vi "LabVIEW 4 MiniGen_Adafruit.vi"(3 "error in (no error)":errorcluster, 4 "dt":dbl=2.65925481e-05 format="%#_9f", 5 "write buffer":string="r512") -> (0 "error out":errorcluster, 1 "Peak Frequency":dbl=514.1242933391554, 2 "magnitude":cluster{"f0":dbl, "df":dbl, "magnitude":dbl[]}={"f0"=146.89265523975868, "df"=73.44632761987934, "magnitude"=[0.0010573193272467023, 0.0008539075571475185, 0.0031903245438082524, 0.016955292518775398, 0.23690823513289183, 0.3602537891013049, 0.13311105968536813, 0.008147783611046596, 0.0029630449976908928, 0.0006136557806143884, 0.0009534776069795952, 0.0014653745421584592, 0.0018598328245117294, 0.000343909019222686, 0.00033893535263468947, 0.0003721335616413998, 0.0003311608729031368, 0.000732767453399492, 0.001587238767052589, 0.0015399953791484678, 0.0006799804044090185, 0.00035922580059501353, 0.00037853640587946584, 0.00040574798016109284, 0.0003944657918505259, 0.00028441301720993916, 0.000261065277392889, 9.830660293093549e-05, 0.00043397339336911814, 0.0005539762634671169, 0.00040990403678268047, 0.00029319183108519875, 8.368304059100074e-05, 8.36004681704598e-05, 0.00015879910796170698, 6.252358099316568e-05, 0.00015881977208714157, 0.00016509561428111567, 6.434491581170871e-05, 0.0001668647295604266, 0.00036578961819133, 0.00045765208783560507, 0.0005154983450355664, 0.0005172148246027255, 0.0003062574513331491, 5.1513455854055797e-05, 0.00023831181783032655, 0.00024374499609663026, 0.0001419110455078641, 0.00041264635419791494, 0.00022761885947105454, 0.00038244224659812054, 0.0003878354411526907, 0.0003434041323071504, 0.00035602580591923087, 0.0003014195763820755, 0.00010701693781615192, 0.00016376183360085065, 0.00021830596775413067, 0.0004512016989735132, 0.00038858135278494886, 0.0003582381020895125, 0.00015397417992981166, 0.00025184195021753214, 0.0003101067745655077, 0.000447806893819167, 0.0006303208430332876, 0.0005244485053927753, 0.0003894931417183425, 0.0002169168936988449, 0.00015424488539364647, 7.28953873783167e-05, 0.00015840874717917624, 0.00030123326854442566, 0.0003357070951253949, 0.0002219813177305886, 2.7096544974727197e-05, 3.534450755456907e-05, 3.428286160556027e-05, 0.00024763168162031965, 0.0005956370452363904, 0.0005001341365814027, 0.0002493340489535057, 8.913553682671315e-05, 4.102695129838161e-05, 0.00023937047150089836, 0.0006064155727417735, 0.0007636718971057465, 0.0005025169233197376, 0.0004592141713891292, 0.0004154038880786475, 0.0004762512230483866, 0.00032394851279825726, 0.00019874656152786516, 0.00024103234975927565, 0.00024679552700484163, 0.00022974190446812425, 0.00014852727721558983, 0.0001534539800413088, 0.0002623950929260538, 0.00020502102196828442, 2.0769438374928514e-05, 3.7831709687521644e-05, 0.00016600027554920273, 7.477285742547296e-05, 0.00015424772258269823, 0.00014615356739457614, 0.0005738937352417223, 0.0005461816457255241, 0.00043653069066669405, 0.00044891438828865895, 0.00033415133284021457, 0.0004333097052614254, 0.0005465034873180447, 0.0004401723358116891, 0.0003491099907256788, 0.00034433390816092396, 0.0001621270437531999, 0.0003023179218436354, 0.000471682669669569, 0.00024159641785356876, 7.693286124485976e-05, 0.0002467093051980444, 0.0003294163904248798, 0.0003712395660317976, 0.00025510195803937145, 0.0002820556822567327, 0.00026127126859739616, 0.0004117321530064503, 0.00026155711305912867, 0.0003954869452259379, 0.0005027179953043017, 0.0002034553573790203, 0.00031739709370906294, 0.000494844481482639, 0.0003194082061686813, 0.00017347199605366486, 0.00030810211276043666, 0.00019142967321880493, 9.299614747889054e-05, 0.00022546314931713994, 0.00024526204479037166, 0.0003803466725698766, 0.0005482171928358633, 0.00022244146310983445, 8.882750051753354e-05, 0.0001521589339551093, 6.025891276057421e-05, 0.00010936756826677184, 0.00011678105621078553, 0.00027208101011661, 0.0003853539959161425, 0.00019733124731021647, 0.0002399298595306906, 0.0003751773029308181, 0.00025934156594460743, 0.0003897060735522648, 0.00028379388433385095, 0.00017344162601981542, 8.946407319767827e-05, 0.0002479505393338664, 0.00027803060344221684, 0.00021717165064423773, 0.0002199029505972962, 0.0004957184252712735, 0.0004894240536570223, 0.0002533586709072349, 0.0001130558253712342, 0.0002151253256980126, 0.00025783922831527315, 8.558793567000533e-05, 0.00023749246624682629, 8.271720418254696e-05, 0.00019562076852570315, 0.00022269512667799665, 0.0002276244107757865, 0.0002727820351925076, 0.00039997710573542355, 0.00032310482776941204, 0.00029355353878777286, 6.098205313979909e-05, 0.0002335475568675092, 0.00016341841260641903, 0.00022823089080733973, 0.0003044010656702124, 0.0001623398261568934, 0.0004701790442476819, 0.0004588133187804099, 0.0006269691947846191, 0.0005404430387144859, 0.00040211372693186285, 0.00019372670536392075, 6.440168512958198e-05, 0.00025538585629209166, 0.0002603927600912937, 0.00025560577048397464, 0.0002262629957829637, 0.0003607957498107714, 0.00030784688204000616, 0.00021197768635284272, 0.0003775437438451099, 0.0002709208729009615, 7.259587758192056e-05, 0.00042224897133781364, 0.0007178070922026255, 0.00047376015823390833, 0.0002390419285937669, 0.00041521474238425424, 0.000549847037281132, 0.00039822948997910514, 0.00044424119183215043, 0.00028924976182143454, 0.000392533131171722, 0.0006030596886870012, 0.00042943037291800384, 0.00015018445254512435, 0.0003089247263095562, 0.00042702952337648293, 0.0003129672107102853, 0.00022654935544524929, 0.00016456577793551, 0.00038796014465995233, 0.00021047618867833676, 0.0002206211444044933, 0.00035334155895193125, 0.00019866739041272719, 0.0002668159983142619, 0.0004925200936011109, 0.00037262502516944185, 0.0003256045216749679, 0.0003440845270831269, 0.0001665288519916862, 0.0001746740042938917, 0.00036685704356912417, 0.0003280980682345908, 0.00026309028815703155, 0.00026930545946579566, 0.000340611458947099, 0.0003731069571000136, 0.0002468870659088116, 0.0002756449502200578, 0.00035429030046231887, 0.0003621555052894118, 0.0003683074149373423, 0.0003306130216987354, 0.00023802697854053423, 8.317737651327105e-05, 0.00015097842581436664, 0.0003288513395746616, 7.503484674742626e-05, 0.00012634741676269078, 6.831559096065801e-05, 0.00020546353367269728, 0.0002085374736113191]} {"magnitude" format="%.2p"; "f0" format="%0.2p"; "df" format="%0.2p"})   [LabVIEW 2020]
uses:
  <vilib>/Instr/_visa.llb/VISA Flush IO Buffer Mask.ctl
  <vilib>/Instr/_visa.llb/VISA Configure Serial Port (Instr).vi
  <vilib>/measure/maspectr.llb/FFT Spectrum (Mag-Phase) for 1 Chan.vi
  <vilib>/measure/NI_MAPro.lvlib
panel:
  in  "Base Freq":dbl=210.0
  out "New Freqency":dbl=11319170.442154845 format="%#_10f"
  in  "N":i32=301
  out "Sample Rate":dbl=37604.51974137822
  out "Waveform Graph":cluster{"f0":dbl, "df":dbl, "magnitude":dbl[]}(graph)={"f0"=146.89265523975868, "df"=73.44632761987934, "magnitude"=[0.0010573193272467023, 0.0008539075571475185, 0.0031903245438082524, 0.016955292518775398, 0.23690823513289183, 0.3602537891013049, 0.13311105968536813, 0.008147783611046596, 0.0029630449976908928, 0.0006136557806143884, 0.0009534776069795952, 0.0014653745421584592, 0.0018598328245117294, 0.000343909019222686, 0.00033893535263468947, 0.0003721335616413998, 0.0003311608729031368, 0.000732767453399492, 0.001587238767052589, 0.0015399953791484678, 0.0006799804044090185, 0.00035922580059501353, 0.00037853640587946584, 0.00040574798016109284, 0.0003944657918505259, 0.00028441301720993916, 0.000261065277392889, 9.830660293093549e-05, 0.00043397339336911814, 0.0005539762634671169, 0.00040990403678268047, 0.00029319183108519875, 8.368304059100074e-05, 8.36004681704598e-05, 0.00015879910796170698, 6.252358099316568e-05, 0.00015881977208714157, 0.00016509561428111567, 6.434491581170871e-05, 0.0001668647295604266, 0.00036578961819133, 0.00045765208783560507, 0.0005154983450355664, 0.0005172148246027255, 0.0003062574513331491, 5.1513455854055797e-05, 0.00023831181783032655, 0.00024374499609663026, 0.0001419110455078641, 0.00041264635419791494, 0.00022761885947105454, 0.00038244224659812054, 0.0003878354411526907, 0.0003434041323071504, 0.00035602580591923087, 0.0003014195763820755, 0.00010701693781615192, 0.00016376183360085065, 0.00021830596775413067, 0.0004512016989735132, 0.00038858135278494886, 0.0003582381020895125, 0.00015397417992981166, 0.00025184195021753214, 0.0003101067745655077, 0.000447806893819167, 0.0006303208430332876, 0.0005244485053927753, 0.0003894931417183425, 0.0002169168936988449, 0.00015424488539364647, 7.28953873783167e-05, 0.00015840874717917624, 0.00030123326854442566, 0.0003357070951253949, 0.0002219813177305886, 2.7096544974727197e-05, 3.534450755456907e-05, 3.428286160556027e-05, 0.00024763168162031965, 0.0005956370452363904, 0.0005001341365814027, 0.0002493340489535057, 8.913553682671315e-05, 4.102695129838161e-05, 0.00023937047150089836, 0.0006064155727417735, 0.0007636718971057465, 0.0005025169233197376, 0.0004592141713891292, 0.0004154038880786475, 0.0004762512230483866, 0.00032394851279825726, 0.00019874656152786516, 0.00024103234975927565, 0.00024679552700484163, 0.00022974190446812425, 0.00014852727721558983, 0.0001534539800413088, 0.0002623950929260538, 0.00020502102196828442, 2.0769438374928514e-05, 3.7831709687521644e-05, 0.00016600027554920273, 7.477285742547296e-05, 0.00015424772258269823, 0.00014615356739457614, 0.0005738937352417223, 0.0005461816457255241, 0.00043653069066669405, 0.00044891438828865895, 0.00033415133284021457, 0.0004333097052614254, 0.0005465034873180447, 0.0004401723358116891, 0.0003491099907256788, 0.00034433390816092396, 0.0001621270437531999, 0.0003023179218436354, 0.000471682669669569, 0.00024159641785356876, 7.693286124485976e-05, 0.0002467093051980444, 0.0003294163904248798, 0.0003712395660317976, 0.00025510195803937145, 0.0002820556822567327, 0.00026127126859739616, 0.0004117321530064503, 0.00026155711305912867, 0.0003954869452259379, 0.0005027179953043017, 0.0002034553573790203, 0.00031739709370906294, 0.000494844481482639, 0.0003194082061686813, 0.00017347199605366486, 0.00030810211276043666, 0.00019142967321880493, 9.299614747889054e-05, 0.00022546314931713994, 0.00024526204479037166, 0.0003803466725698766, 0.0005482171928358633, 0.00022244146310983445, 8.882750051753354e-05, 0.0001521589339551093, 6.025891276057421e-05, 0.00010936756826677184, 0.00011678105621078553, 0.00027208101011661, 0.0003853539959161425, 0.00019733124731021647, 0.0002399298595306906, 0.0003751773029308181, 0.00025934156594460743, 0.0003897060735522648, 0.00028379388433385095, 0.00017344162601981542, 8.946407319767827e-05, 0.0002479505393338664, 0.00027803060344221684, 0.00021717165064423773, 0.0002199029505972962, 0.0004957184252712735, 0.0004894240536570223, 0.0002533586709072349, 0.0001130558253712342, 0.0002151253256980126, 0.00025783922831527315, 8.558793567000533e-05, 0.00023749246624682629, 8.271720418254696e-05, 0.00019562076852570315, 0.00022269512667799665, 0.0002276244107757865, 0.0002727820351925076, 0.00039997710573542355, 0.00032310482776941204, 0.00029355353878777286, 6.098205313979909e-05, 0.0002335475568675092, 0.00016341841260641903, 0.00022823089080733973, 0.0003044010656702124, 0.0001623398261568934, 0.0004701790442476819, 0.0004588133187804099, 0.0006269691947846191, 0.0005404430387144859, 0.00040211372693186285, 0.00019372670536392075, 6.440168512958198e-05, 0.00025538585629209166, 0.0002603927600912937, 0.00025560577048397464, 0.0002262629957829637, 0.0003607957498107714, 0.00030784688204000616, 0.00021197768635284272, 0.0003775437438451099, 0.0002709208729009615, 7.259587758192056e-05, 0.00042224897133781364, 0.0007178070922026255, 0.00047376015823390833, 0.0002390419285937669, 0.00041521474238425424, 0.000549847037281132, 0.00039822948997910514, 0.00044424119183215043, 0.00028924976182143454, 0.000392533131171722, 0.0006030596886870012, 0.00042943037291800384, 0.00015018445254512435, 0.0003089247263095562, 0.00042702952337648293, 0.0003129672107102853, 0.00022654935544524929, 0.00016456577793551, 0.00038796014465995233, 0.00021047618867833676, 0.0002206211444044933, 0.00035334155895193125, 0.00019866739041272719, 0.0002668159983142619, 0.0004925200936011109, 0.00037262502516944185, 0.0003256045216749679, 0.0003440845270831269, 0.0001665288519916862, 0.0001746740042938917, 0.00036685704356912417, 0.0003280980682345908, 0.00026309028815703155, 0.00026930545946579566, 0.000340611458947099, 0.0003731069571000136, 0.0002468870659088116, 0.0002756449502200578, 0.00035429030046231887, 0.0003621555052894118, 0.0003683074149373423, 0.0003306130216987354, 0.00023802697854053423, 8.317737651327105e-05, 0.00015097842581436664, 0.0003288513395746616, 7.503484674742626e-05, 0.00012634741676269078, 6.831559096065801e-05, 0.00020546353367269728, 0.0002085374736113191]}
  in  "VISA resource name":refnum<visa-resource-name>="COM12"
  out "read buffer":string="Output = 2500,2454,2418,2378,2328,2280,2224,2162,2104,2066,2008,1948,1896,1840,1788,1742,1694,1660,1616,1584,1540,1510,1486,1468,1448,1438,1426,1422,1428,1420,1432,1456,1468,1486,1504,1548,1582,1620,1648,1702,1748,1788,1850,1896,1954,1988,2044,2110,2170,2218,2272,2320,2368,2412,2468,2506,2530,2576,2598,2628,2662,2676,2684,2698,2712,2714,2716,2710,2694,2684,2664,2644,2618,2580,2558,2510,2472,2432,2388,2334,2288,2226,2186,2124,2076,2014,1960,1916,1860,1808,1764,1706,1670,1630,1590,1556,1520,1492,1476,1450,1448,1426,1418,1426,1424,1430,1442,1468,1482,1506,1540,1572,1602,1644,1690,1736,1788,1836,1886,1934,1996,2044,2096,2150,2210,2260,2304,2354,2410,2454,2500,2530,2568,2598,2628,2660,2666,2694,2694,2710,2710,2704,2710,2694,2674,2656,2644,2612,2590,2556,2510,2476,2426,2382,2344,2290,2238,2186,2130,2082,2010,1956,1916,1852,1814,1754,1718,1672,1628,1596,1562,1520,1496,1478,1460,1446,1432,1424,1428,1414,1432,1452,1456,1474,1504,1538,1558,1600,1638,1682,1726,1774,1828,1870,1916,1966,2030,2090,2138,2192,2254,2288,2348,2384,2436,2488,2516,2550,2592,2626,2650,2664,2684,2700,2706,2716,2714,2704,2694,2680,2664,2656,2626,2600,2570,2528,2484,2452,2398,2362,2306,2260,2206,2144,2100,2042,1986,1942,1878,1830,1776,1722,1686,1632,1606,1570,1536,1500,1482,1466,1442,1430,1430,1414,1428,1428,1444,1454,1474,1498,1512,1564,1582,1620,1652,1706,1760,1810,1862,1902,1960,2022,2082,2134,2186,2238,2288,2342,2388,2428,2480,2522,2548,2592,2622,2648,2660,2674,2686,2712,2714,2718,2702,2694,2696,2672,2648,2628,2612,2572,2532,2500,2460,2422,2372,2320,2272,2218,2162,2106,2048,1998,1942,1886,1830,1776,1740,1690,1650,1614,1572,1546,1502,1490,1460,1444,1434,1426,1426,1428,1424,1436,1456,1462,1488,1522,1556,1578,1624,1664,1712,1758,1796,1848,1900,1950,2014,2072,2116,2182,2234,2278,2334,2374,2434,2472,2514,2552,2582,2618,2634,2660,2674,2688,2696,2700,2718,2704,2706,2694,2668,2658,2636,2604,2566,2534,2494,2466,2420,2370,2314,2264,2218,2172,2106,2062,1998,1948,1898,1848,1794,1742,1696,1650,1616,1574,1546,1514,1486,1464,1452,1440,1424,1420,1416,1432,1440,1448,1464,1482,1518,1542,1580,1612,1652,1706,1748,1806,1856,1894,1958,2010,2062,2116,2180,2232,2286,2330,2384,2428,2474,2510,2554,2588,2616,2640,2666,2680,2684,2698,2716,2708,2712,2706,2694,2676,2648,2624,2604,2578,2538,2492,2460,2414,2368,2326,2266,2206,2158,2104,2062,1992,1940,1892,1838,1792,1736,1700,1652,1616,1578,1546,1518,1492,1454,1454,1428,1432,1432,1412,1430,1434,1444,1472,1494,1522,1550,1574,1620,1662,1696,1748,1796,1852,1900,1950,2004,2062,2122,2174,2226,2274,2328,2372,2416,2462,2506,2548,2584,2604,2638,2660\r\n"
  out "XY Graph":cluster{dbl[], dbl[]}[](graph)
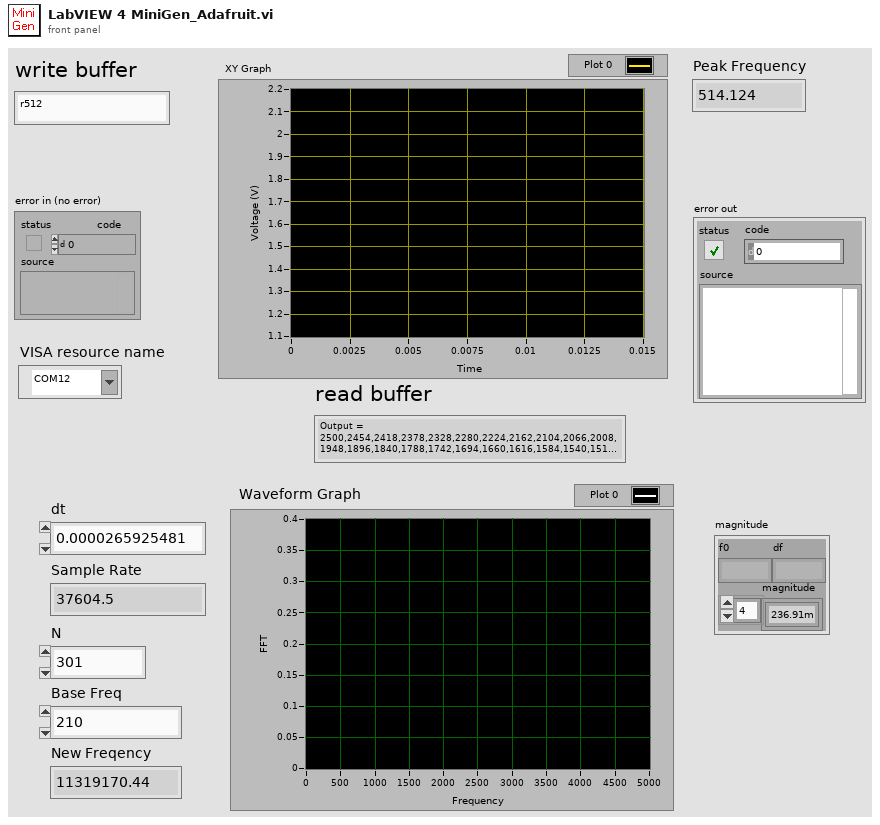
[diagram p1: front panel]
types:
  T1 = typedef "VISA Flush IO Buffer Mask.ctl" = u16
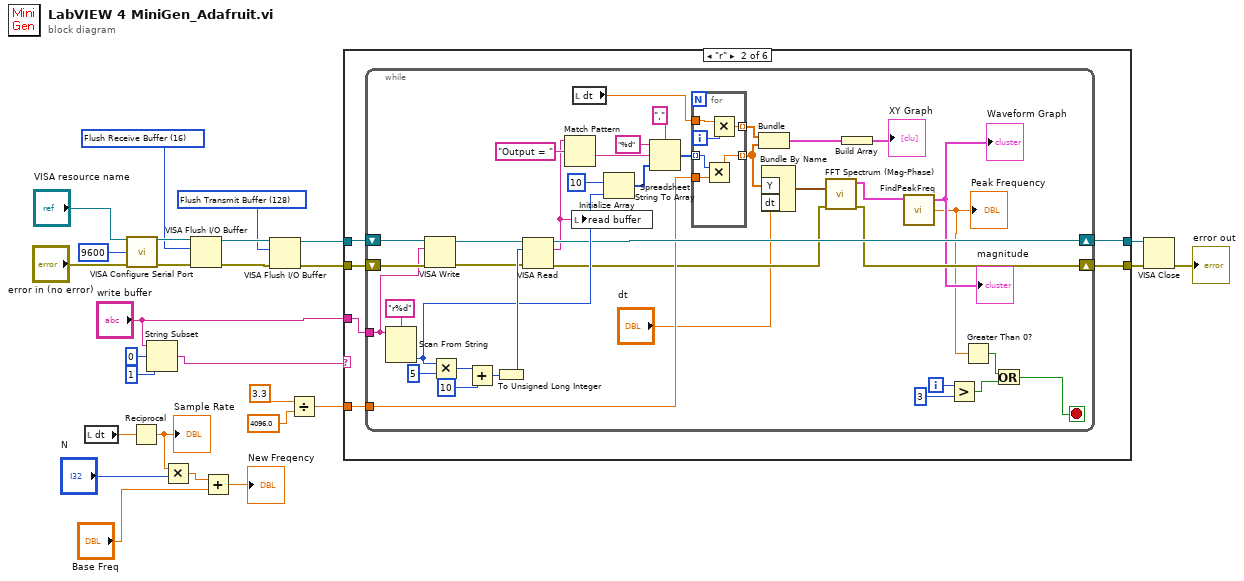
[diagram p0: block diagram]
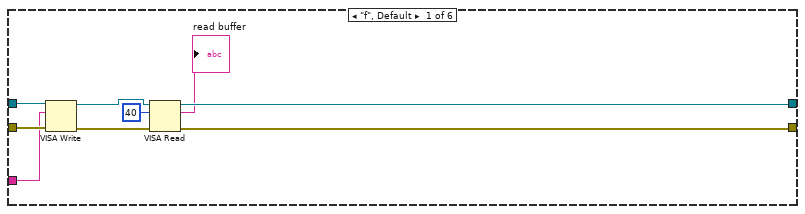
[diagram p2: hidden frame]
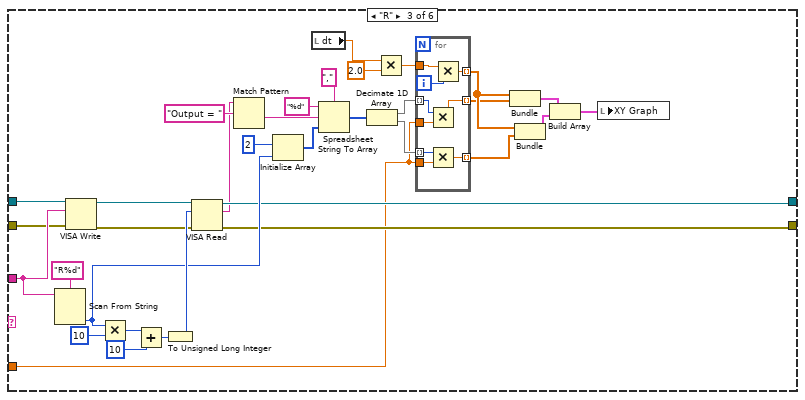
[diagram p3: hidden frame]
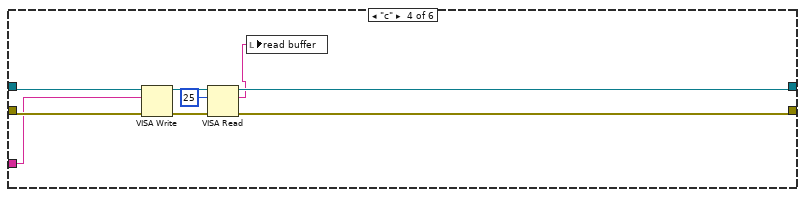
[diagram p4: hidden frame]
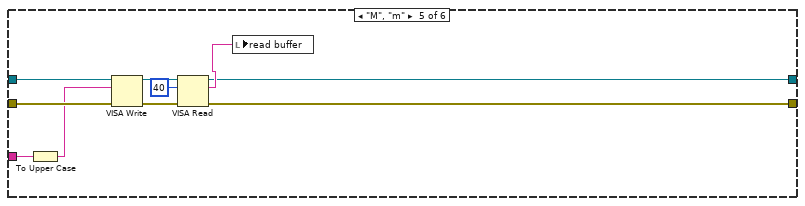
[diagram p5: hidden frame]
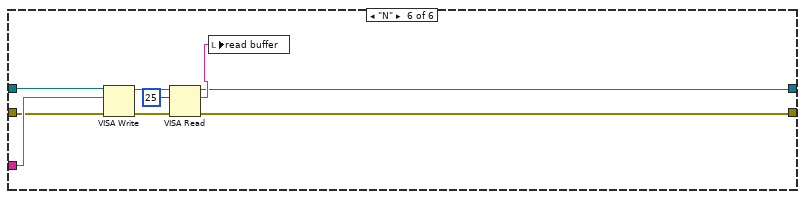
[diagram p6: hidden frame]
diagram:
  w21 = T1 128 items=["Flush Receive Buffer"=16, "Write Transmit Buffer to Device"=32, "Flush Receive Buffer (No I/O)"=64, "Flush Transmit Buffer"=128] ("Mask")
  w24 = T1 16 items=["Flush Receive Buffer"=16, "Write Transmit Buffer to Device"=32, "Flush Receive Buffer (No I/O)"=64, "Flush Transmit Buffer"=128] ("Mask")
  n1 = local read "dt"() -> (w8:dbl)
  n2 = call-poly "VISA Configure Serial Port"("VISA resource name"="VISA resource name", "baud rate (9600)"=u32 9600, "error in (no error)"="error in (no error)") -> ("VISA resource name out"=w26:refnum<visa-resource-name>, "error out"=w25:errorcluster)  [unwired: 11 in]
  n3 = Reciprocal(x=w8) -> (1/x=w7:dbl)
  "Sample Rate" <- w7
  n4 = String Subset(string="write buffer", offset (0)=0, length (rest)=1 ("length (rest)")) -> (substring=w14:string)
  n5 = Multiply(x=w7, y="N") -> (x*y=w5:dbl)
  n6 = VISA Flush I/O Buffer(VISA resource name=w26, mask (16)=w24, error in (no error)=w25) -> (VISA resource name out=w23:refnum<visa-resource-name>, error out=w22:errorcluster)
  n7 = Add(x=w5, y="Base Freq") -> (x+y=→"New Freqency":dbl)
  n8 = VISA Flush I/O Buffer(VISA resource name=w23, mask (16)=w21, error in (no error)=w22) -> (VISA resource name out=w2:refnum<visa-resource-name>, error out=w1:errorcluster)
  n9 = Divide(x=3.3, y=4096.0) -> (x/y=w9:dbl)
  n10 = case shown="\"r\"" w14 {
    tunnel: [w36 w37 w106 w133 w140 w150] -> w20
    tunnel: [w34 w39 w107 w134 w141 w151] -> w19
    tunnel: w2 -> [w32 w41 w95 w136 w145 w154]
    tunnel: w1 -> [w31 w40 w93 w135 w144 w152]
    tunnel: "write buffer" -> [w28 w42 w94 w132 w143 w153]
    tunnel: w9 -> [_ w38 w98 _ _ _]
    frame "f", Default {
      n11 = VISA Write(VISA resource name=w32, write buffer=w28, error in (no error)=w31) -> (VISA resource name out=w29:refnum<visa-resource-name>, error out=w30:errorcluster)  [unwired: 1 out]
      n12 = VISA Read(VISA resource name=w29, byte count=u32 40, error in (no error)=w30) -> (VISA resource name out=w34:refnum<visa-resource-name>, read buffer=→"read buffer":string, error out=w36:errorcluster)  [unwired: 1 out]
    }
    frame "r" {
      n13 = while {
        tunnel: w42 -> [w50]
        tunnel: w38 -> [w63]
        shift-right: [w64] -> w39
        shift-left: w41 -> [w54]
        shift-right: [w60] -> w37
        shift-left: w40 -> [w53]
        i -> [w48]
        stop <- w44 stop-if-true
        n14 = Scan From String(format string="r%d", input string=w50) -> (output 1=w70:i32)  [unwired: 3 in, 3 out]
        n15 = VISA Write(VISA resource name=w54, write buffer=w50, error in (no error)=w53) -> (VISA resource name out=w51:refnum<visa-resource-name>, error out=w52:errorcluster)  [unwired: 1 out]
        n16 = Multiply(x=w70, y=5) -> (x*y=w79:i32)
        n17 = Add(x=w79, y=10) -> (x+y=w77:i32)
        n18 = To Unsigned Long Integer(number=w77) -> (unsigned 32bit integer=w76:u32)
        n19 = VISA Read(VISA resource name=w51, byte count=w76, error in (no error)=w52) -> (VISA resource name out=w64:refnum<visa-resource-name>, read buffer=w43:string, error out=w61:errorcluster)  [unwired: 1 out]
        n20 = Match Pattern(string=w43, regular expression="Output = ") -> (after substring=w74:string)  [unwired: 1 in, 3 out]
        n21 = local write "read buffer"(w43) -> ()
        n22 = local read "dt"() -> (w58:dbl)
        n23 = Initialize Array(10 ("y"), w70) -> (w69:i32[])
        n24 = Spreadsheet String To Array(delimiter (Tab)=",", format string="%d", spreadsheet string=w74, array type (2D Dbl)=w69) -> (array=w68:i32[])
        n25 = for {
          tunnel: w68 -> [w87] mode=indexing
          tunnel: [w85] -> w57 mode=indexing
          tunnel: [w82] -> w67 mode=indexing
          tunnel: w63 -> [w86]
          tunnel: w58 -> [w83]
          i -> [w84]
          n26 = Multiply(x=w87, y=w86) -> (x*y=w85:dbl)
          n27 = Multiply(x=w83, y=w84) -> (x*y=w82:dbl)
        }
        n28 = Bundle(w67, w57) -> (w66:cluster{dbl[], dbl[]})  [unwired: 1 in]
        n29 = Bundle By Name("Y"=w57, "dt"="dt") -> (w62:waveform(dbl))  [unwired: 1 in]
        n30 = call-poly <vilib>:"FFT Spectrum (Mag-Phase).vi"("error in (no error)"=w61, "time signal"=w62) -> ("error out"=w60:errorcluster, "magnitude"=w56:cluster{"f0":dbl, "df":dbl, "magnitude":dbl[]})  [unwired: 5 in, 3 out]
        n31 = Build Array(w66) -> (→"XY Graph":cluster{dbl[], dbl[]}[])
        n32 = call "FindPeakFreq.vi"("magnitude"=w56) -> ("Max"=w49:dbl, "output cluster"=→"Waveform Graph" →"magnitude":cluster{"f0":dbl, "df":dbl, "magnitude":dbl[]})  [unwired: 3 in]
        "Peak Frequency" <- w49
        n33 = Greater?(x=w48, y=3) -> (0:w46:bool)
        n34 = Greater Than 0?(x=w49) -> (x > 0?=w45:bool)
        n35 = Or(x=w45, y=w46) -> (x .or. y?=w44:bool)
      }
    }
    frame "R" {
      n36 = Scan From String(format string="R%d", input string=w94) -> (output 1=w109:i32)  [unwired: 3 in, 3 out]
      n37 = VISA Write(VISA resource name=w95, write buffer=w94, error in (no error)=w93) -> (VISA resource name out=w92:refnum<visa-resource-name>, error out=w91:errorcluster)  [unwired: 1 out]
      n38 = Multiply(x=w109, y=10) -> (x*y=w119:i32)
      n39 = Add(x=w119, y=10) -> (x+y=w117:i32)
      n40 = To Unsigned Long Integer(number=w117) -> (unsigned 32bit integer=w116:u32)
      n41 = VISA Read(VISA resource name=w92, byte count=w116, error in (no error)=w91) -> (VISA resource name out=w107:refnum<visa-resource-name>, read buffer=w96:string, error out=w106:errorcluster)  [unwired: 1 out]
      n42 = Match Pattern(string=w96, regular expression="Output = ") -> (after substring=w114:string)  [unwired: 1 in, 3 out]
      n43 = Initialize Array(2 ("y"), w109) -> (w111:i32[])
      n44 = local read "dt"() -> (w89:dbl)
      n45 = Spreadsheet String To Array(delimiter (Tab)=",", format string="%d", spreadsheet string=w114, array type (2D Dbl)=w111) -> (array=w108:i32[])
      n46 = Decimate 1D Array(w108) -> (w105:i32[], w104:i32[])
      n47 = Multiply(x=w89, y=2.0) -> (x*y=w90:dbl)
      n48 = for {
        tunnel: w105 -> [w130] mode=indexing
        tunnel: [w128] -> w100 mode=indexing
        tunnel: [w125] -> w101 mode=indexing
        tunnel: w98 -> [w129]
        tunnel: w90 -> [w126]
        tunnel: w104 -> [w124] mode=indexing
        tunnel: [w123] -> w99 mode=indexing
        tunnel: w98 -> [w122]
        i -> [w127]
        n49 = Multiply(x=w130, y=w129) -> (x*y=w128:dbl)
        n50 = Multiply(x=w124, y=w122) -> (x*y=w123:dbl)
        n51 = Multiply(x=w126, y=w127) -> (x*y=w125:dbl)
      }
      n52 = Bundle(w101, w100) -> (w102:cluster{dbl[], dbl[]})  [unwired: 1 in]
      n53 = Bundle(w101, w99) -> (w103:cluster{dbl[], dbl[]})  [unwired: 1 in]
      n54 = Build Array(w102, w103) -> (w97:cluster{dbl[], dbl[]}[])
      n55 = local write "XY Graph"(w97) -> ()
    }
    frame "c" {
      n56 = VISA Write(VISA resource name=w136, write buffer=w132, error in (no error)=w135) -> (VISA resource name out=w139:refnum<visa-resource-name>, error out=w138:errorcluster)  [unwired: 1 out]
      n57 = VISA Read(VISA resource name=w139, byte count=u32 25, error in (no error)=w138) -> (VISA resource name out=w134:refnum<visa-resource-name>, read buffer=w131:string, error out=w133:errorcluster)  [unwired: 1 out]
      n58 = local write "read buffer"(w131) -> ()
    }
    frame "M", "m" {
      n59 = To Upper Case(1:w143) -> (0:w142:string)
      n60 = VISA Write(VISA resource name=w145, write buffer=w142, error in (no error)=w144) -> (VISA resource name out=w148:refnum<visa-resource-name>, error out=w149:errorcluster)  [unwired: 1 out]
      n61 = VISA Read(VISA resource name=w148, byte count=u32 40, error in (no error)=w149) -> (VISA resource name out=w141:refnum<visa-resource-name>, read buffer=w146:string, error out=w140:errorcluster)  [unwired: 1 out]
      n62 = local write "read buffer"(w146) -> ()
    }
    frame "N" {
      n63 = VISA Write(VISA resource name=w154, write buffer=w153, error in (no error)=w152) -> (VISA resource name out=w158:refnum<visa-resource-name>, error out=w157:errorcluster)  [unwired: 1 out]
      n64 = VISA Read(VISA resource name=w158, byte count=u32 25, error in (no error)=w157) -> (VISA resource name out=w151:refnum<visa-resource-name>, read buffer=w156:string, error out=w150:errorcluster)  [unwired: 1 out]
      n65 = local write "read buffer"(w156) -> ()
    }
  }
  n66 = VISA Close(VISA resource name=w19, error in (no error)=w20) -> (error out=→"error out":errorcluster)
